vi "New VI.vi"() -> ()   [LabVIEW 2016]
panel:
  in  "Boolean":bool
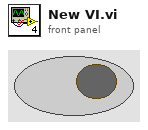
[diagram p1: front panel]
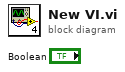
[diagram p0: block diagram]
diagram:
